vi "Update State on Cursor Move.vi"(9 "Cursor.Position.X":dbl, 10 "Cursor Name":string, 11 "Display State In":T1 caption="State") -> (2 "cursor type":string, 3 "Display State out":T1 caption="State")   [LabVIEW 2017, in "Waveforms with Cursors.xctl"]
uses:
  <vilib>/addons/_XControls/Waveforms with Cursors/Waveforms with Cursors.xctl
  <vilib>/addons/_XControls/Waveforms with Cursors/Controls/State.ctl
  <vilib>/Utility/miscctls.llb/LVFontTypeDef.ctl
  <vilib>/addons/_XControls/Waveforms with Cursors/Controls/Waveform Cursor Configuration.ctl
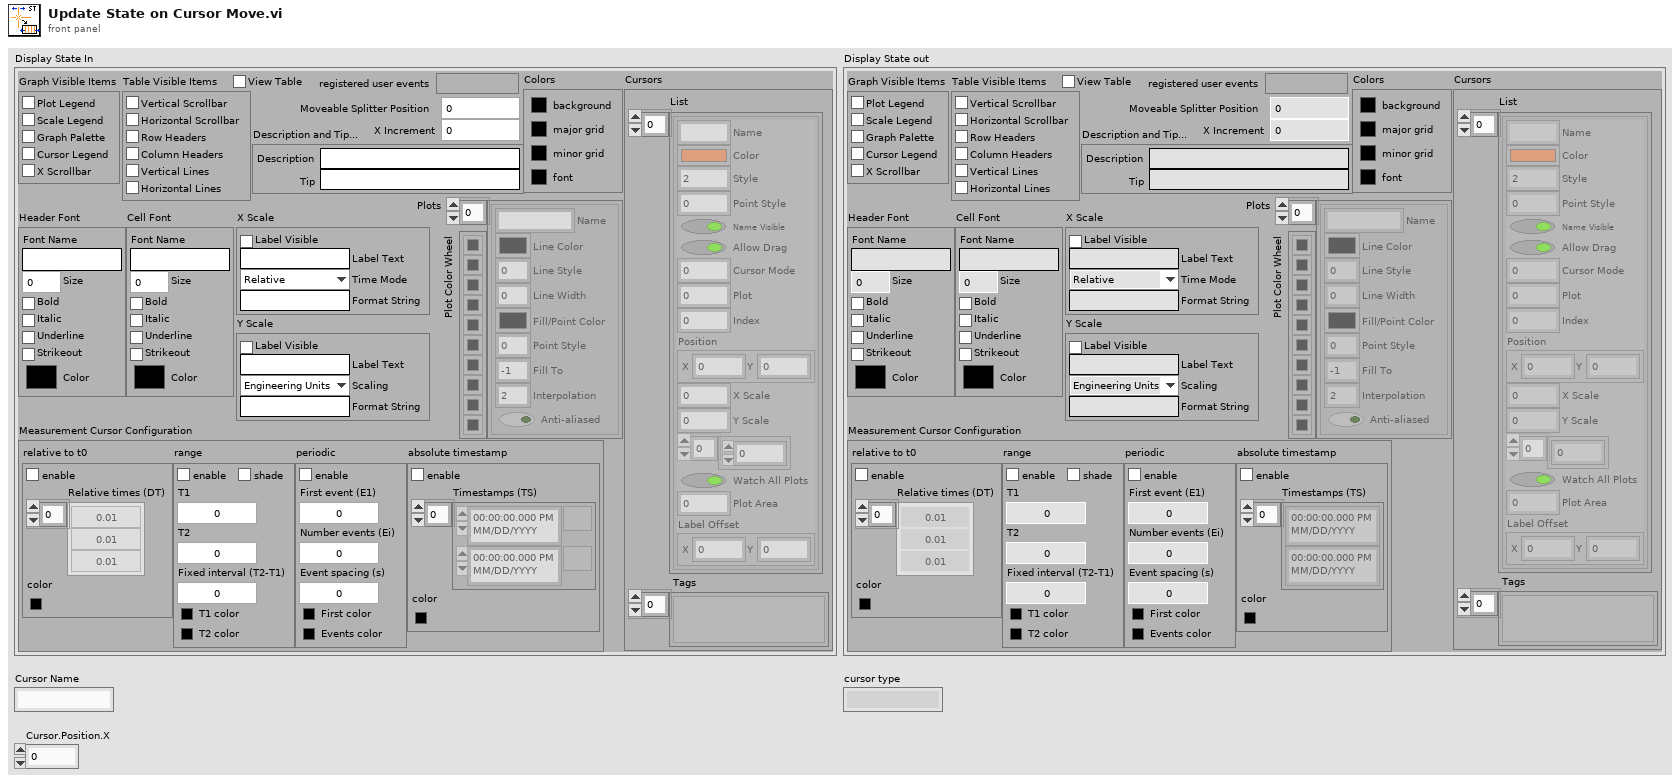
[diagram p1: front panel]
types:
  T1 = typedef "Waveforms with Cursors.xctl/State.ctl" = cluster{"Graph Visible Items":cluster{"Plot Legend":bool, "Scale Legend":bool, "Graph Palette":bool, "Cursor Legend":bool, "X Scrollbar":bool}, "View Table":bool, "Table Visible Items":cluster{"Vertical Scrollbar":bool, "Horizontal Scrollbar":bool, "Row Headers":bool, "Column Headers":bool, "Vertical Lines":bool, "Horizontal Lines":bool}, "Header Font":T2, "Cell Font":T2, "Description and Tip...":cluster{"Description":string, "Tip":string}, "Moveable Splitter Position":i32, "Measurement Cursor Configuration":T3, "X Increment":dbl, "X Scale":cluster{"Label Visible":bool, "Label Text":string, "Time Mode":enum16{"Relative", "Absolute"}, "Format String":string}, "Y Scale":cluster{"Label Visible":bool, "Label Text":string, "Scaling":enum16{"Engineering Units", "Voltage"}, "Format String":string}, "Colors":cluster{"background":u32, "major grid":u32, "minor grid":u32, "font":u32}, "Cursors":cluster{"List":cluster{"Name":string, "Color":u32, "Style":i32, "Point Style":u8, "Name Visible":bool, "Allow Drag":bool, "Cursor Mode":u32, "Plot":i32, "Index":i32, "Position":cluster{"X":dbl, "Y":dbl}, "X Scale":u32, "Y Scale":u32, "Watch Plots":i32[], "Watch All Plots":bool, "Plot Area":i32, "Label Offset":cluster{"X":dbl, "Y":dbl}}[], "Tags":variant[]}, "Plots":cluster{"Name":string, "Line Color":u32, "Line Style":u8, "Line Width":u8, "Fill/Point Color":u32, "Point Style":u8, "Fill To":i16, "Interpolation":u8, "Anti-aliased":bool}[], "Plot Color Wheel":u32[], "registered user events":variant}
  T2 = typedef "LVFontTypeDef.ctl" = cluster{"Font Name":string, "Size":u16, "Bold":bool, "Italic":bool, "Underline":bool, "Strikeout":bool, "Color":u32}
  T3 = typedef "Waveforms with Cursors.xctl/Waveform Cursor Configuration.ctl" = cluster{"relative to t0":cluster{"enable relative time":bool, "Relative times (DT)":dbl[], "color":u32}, "range":cluster{"enable range":bool, "T1":dbl, "T2":dbl, "Fixed interval (T2-T1)":dbl, "T1 color":u32, "T2 color":u32, "enable shading":bool}, "periodic":cluster{"enable periodic":bool, "First event (E1)":dbl, "Number events (Ei)":i32, "Event spacing (s)":dbl, "First color":u32, "Events color":u32}, "absolute timestamp":cluster{"enable absolute":bool, "Timestamps (TS)":timestamp[], "color":u32}}
  T4 = cluster{"Name":string, "Color":u32, "Style":i32, "Point Style":u8, "Name Visible":bool, "Allow Drag":bool, "Cursor Mode":u32, "Plot":i32, "Index":i32, "Position":cluster{"X":dbl, "Y":dbl}, "X Scale":u32, "Y Scale":u32, "Watch Plots":i32[], "Watch All Plots":bool, "Plot Area":i32, "Label Offset":cluster{"X":dbl, "Y":dbl}}[]
  T5 = cluster{"Name":string, "Color":u32, "Style":i32, "Point Style":u8, "Name Visible":bool, "Allow Drag":bool, "Cursor Mode":u32, "Plot":i32, "Index":i32, "Position":cluster{"X":dbl, "Y":dbl}, "X Scale":u32, "Y Scale":u32, "Watch Plots":i32[], "Watch All Plots":bool, "Plot Area":i32, "Label Offset":cluster{"X":dbl, "Y":dbl}}
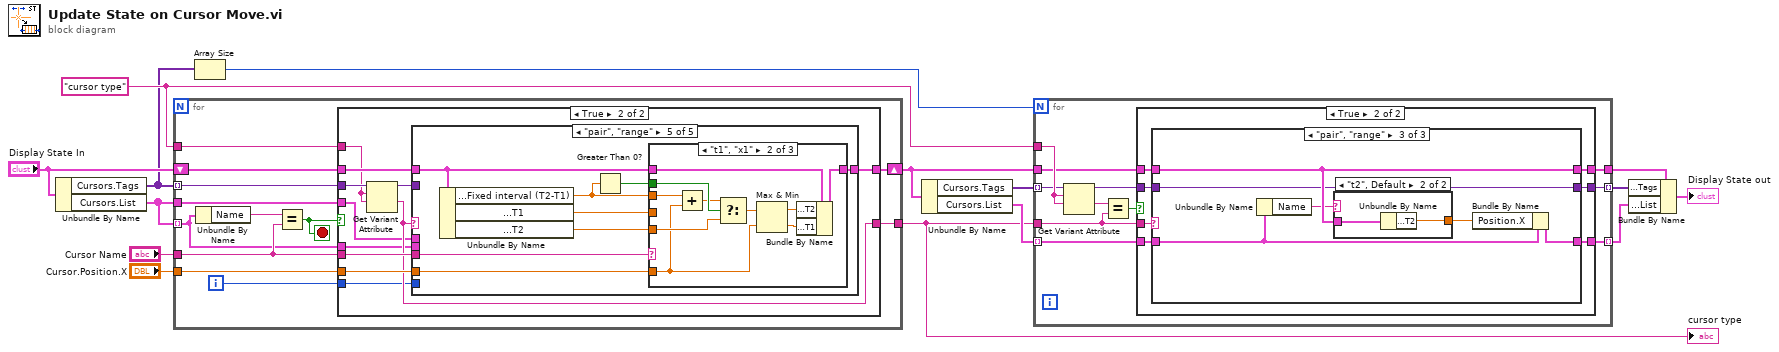
[diagram p0: block diagram]
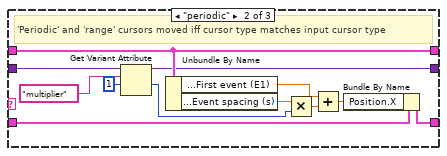
[diagram p4: hidden frame]
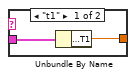
[diagram p5: hidden frame]
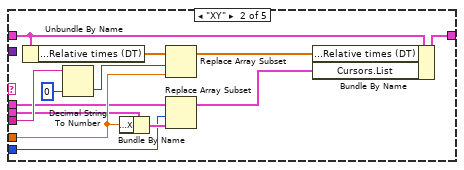
[diagram p8: hidden frame]
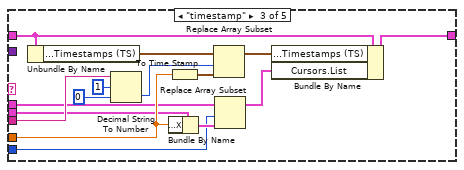
[diagram p9: hidden frame]
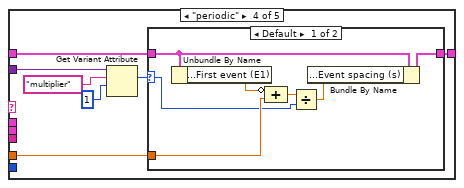
[diagram p10: hidden frame]
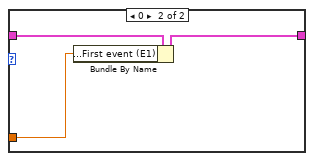
[diagram p11: hidden frame]
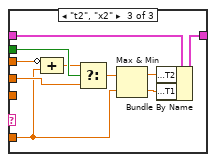
[diagram p13: hidden frame]
diagram:
  w12 = "cursor type"
  n1 = Unbundle By Name("Display State In") -> ("Cursors.Tags"=w2:variant[], "Cursors.List"=w4:T4)
  n2 = for {
    tunnel: "Cursor Name" -> [w24]
    tunnel: "Cursor.Position.X" -> [w25]
    shift-right: [w26] -> w14
    shift-left: "Display State In" -> [w27]
    tunnel: [w23] -> w5
    tunnel: w12 -> [w22]
    tunnel: w2 -> [w21] mode=indexing
    tunnel: w4 -> [w18] mode=indexing
    tunnel: w4 -> [w19]
    i -> [w17]
    stop <- w16 stop-if-true
    n3 = Unbundle By Name(w18) -> ("Name"=w20:string)
    n4 = Equal?(x=w20, y=w24) -> (x = y?=w16:bool)
    n5 = case shown="True" w16 {
      tunnel: w21 -> [_ w39]
      tunnel: w22 -> [_ w32]
      tunnel: w27 -> [w28 w38]
      tunnel: [w28 w37] -> w26
      tunnel: w25 -> [_ w35]
      tunnel: w24 -> [_ w34]
      tunnel: [_ w33] -> w23
      tunnel: w19 -> [_ w31]
      tunnel: w18 -> [_ w30]
      tunnel: w17 -> [_ w29]
      frame False {
      }
      frame True {
        n6 = Get Variant Attribute(Variant=w39, name=w32, default value (empty Variant)=w32) -> (duplicate Variant=w36:variant, value=w33:string)  [unwired: 1 in, 2 out]
        n7 = case shown="\"pair\", \"range\"" w33 {
          tunnel: w38 -> [w40 w51 w66 w75 w91]
          tunnel: [w40 w53 w68 w74 w93] -> w37
          tunnel: w36 -> [_ _ _ w73 _]
          tunnel: w35 -> [_ w46 w58 w70 w92]
          tunnel: w34 -> [_ w47 w62 _ w90]
          tunnel: w31 -> [_ w44 w56 _ _]
          tunnel: w30 -> [_ w45 w57 _ _]
          tunnel: w29 -> [_ w42 w55 _ _]
          frame Default {
          }
          frame "XY" {
            n8 = Unbundle By Name(w51) -> ("Measurement Cursor Configuration.relative to t0.Relative times (DT)"=w50:dbl[])
            n9 = Decimal String To Number(string=w47, default (0L)=0 ("default (0 I32)")) -> (number=w49:i32)  [unwired: 1 in, 1 out]
            n10 = Bundle By Name(cluster=w45, "Position.X"=w46) -> (w43:T5)
            n11 = Replace Array Subset(array=w50, new element=w46, index=w49) -> (w48:dbl[])
            n12 = Replace Array Subset(array=w44, new element=w43, index=w42) -> (w41:T4)
            n13 = Bundle By Name(cluster=w51, "Measurement Cursor Configuration.relative to t0.Relative times (DT)"=w48, "Cursors.List"=w41) -> (w53:T1)
          }
          frame "timestamp" {
            n14 = Unbundle By Name(w66) -> ("Measurement Cursor Configuration.absolute timestamp.Timestamps (TS)"=w65:timestamp[])
            n15 = Decimal String To Number(string=w62, offset=1, default (0L)=0 ("default (0 I32)")) -> (number=w64:i32)  [unwired: 1 out]
            n16 = Bundle By Name(cluster=w57, "Position.X"=w58) -> (w59:T5)
            n17 = To Time Stamp(1:w58) -> (0:w61:timestamp)
            n18 = Replace Array Subset(array=w65, new element=w61, index=w64) -> (w63:timestamp[])
            n19 = Replace Array Subset(array=w56, new element=w59, index=w55) -> (w54:T4)
            n20 = Bundle By Name(cluster=w66, "Measurement Cursor Configuration.absolute timestamp.Timestamps (TS)"=w63, "Cursors.List"=w54) -> (w68:T1)
          }
          frame "periodic" {
            n21 = Get Variant Attribute(Variant=w73, name="multiplier", default value (empty Variant)=1) -> (value=w69:i32)  [unwired: 1 in, 3 out]
            n22 = case shown="Default" w69 {
              selector: w69 -> [w78 _]
              tunnel: w75 -> [w81 w85]
              tunnel: [w82 w84] -> w74
              tunnel: w70 -> [w79 w83]
              frame Default {
                n23 = Unbundle By Name(w81) -> ("Measurement Cursor Configuration.periodic.First event (E1)"=w80:dbl)
                n24 = Compound Arithmetic op=ADD(invert w80, w79) -> (w77:dbl)
                n25 = Divide(x=w77, y=w78) -> (x/y=w76:dbl)
                n26 = Bundle By Name(cluster=w81, "Measurement Cursor Configuration.periodic.Event spacing (s)"=w76) -> (w82:T1)
              }
              frame 0 {
                n27 = Bundle By Name(cluster=w85, "Measurement Cursor Configuration.periodic.First event (E1)"=w83) -> (w84:T1)
              }
            }
          }
          frame "pair", "range" {
            n28 = Unbundle By Name(w91) -> ("Measurement Cursor Configuration.range.Fixed interval (T2-T1)"=w86:dbl, "Measurement Cursor Configuration.range.T1"=w89:dbl, "Measurement Cursor Configuration.range.T2"=w88:dbl)
            n29 = Greater Than 0?(x=w86) -> (x > 0?=w87:bool)
            n30 = case shown="\"t1\", \"x1\"" w90 {
              tunnel: w91 -> [w94 w104 w114]
              tunnel: [w94 w103 w113] -> w93
              tunnel: w92 -> [_ w97 w105]
              tunnel: w89 -> [_ _ w106]
              tunnel: w88 -> [_ w99 _]
              tunnel: w86 -> [_ w101 w111]
              tunnel: w87 -> [_ w102 w112]
              frame Default {
              }
              frame "t1", "x1" {
                n31 = Add(x=w101, y=w97) -> (x+y=w100:dbl)
                n32 = Select(t=w100, s=w102, f=w99) -> (s? t:f=w98:dbl)
                n33 = Max & Min(x=w98, y=w97) -> (max(x,y)=w96:dbl, min(x,y)=w95:dbl)
                n34 = Bundle By Name(cluster=w104, "Measurement Cursor Configuration.range.T2"=w96, "Measurement Cursor Configuration.range.T1"=w95) -> (w103:T1)
              }
              frame "t2", "x2" {
                n35 = Compound Arithmetic op=ADD(invert w111, w105) -> (w110:dbl)
                n36 = Select(t=w110, s=w112, f=w106) -> (s? t:f=w109:dbl)
                n37 = Max & Min(x=w109, y=w105) -> (max(x,y)=w108:dbl, min(x,y)=w107:dbl)
                n38 = Bundle By Name(cluster=w114, "Measurement Cursor Configuration.range.T2"=w108, "Measurement Cursor Configuration.range.T1"=w107) -> (w113:T1)
              }
            }
          }
        }
      }
    }
  }
  "cursor type" <- w5
  n39 = Array Size(array=w2) -> (size(s)=w3:i32)
  n40 = Unbundle By Name(w14) -> ("Cursors.Tags"=w6:variant[], "Cursors.List"=w7:T4)
  n41 = for {
    N: w3 -> [_]
    tunnel: w12 -> [w125]
    tunnel: w5 -> [w121]
    tunnel: w6 -> [w119] mode=indexing
    tunnel: w7 -> [w118] mode=indexing
    tunnel: w14 -> [w120]
    tunnel: [w117] -> w8 mode=indexing
    tunnel: [w116] -> w9 mode=indexing
    tunnel: [w115] -> w10
    n42 = Get Variant Attribute(Variant=w119, name=w125, default value (empty Variant)=w125) -> (duplicate Variant=w124:variant, value=w122:string)  [unwired: 1 in, 2 out]
    n43 = Equal?(x=w122, y=w121) -> (x = y?=w123:bool)
    n44 = case shown="True" w123 {
      tunnel: w124 -> [w127 w133]
      tunnel: w120 -> [w128 w135]
      tunnel: w121 -> [_ w134]
      tunnel: [w128 w132] -> w115
      tunnel: w118 -> [w126 w131]
      tunnel: [w126 w130] -> w117
      tunnel: [w127 w129] -> w116
      frame False {
      }
      frame True {
        n45 = case shown="\"pair\", \"range\"" w134 {
          tunnel: w135 -> [w138 w141 w156]
          tunnel: w133 -> [w137 w150 w155]
          tunnel: [w138 w141 w156] -> w132
          tunnel: w131 -> [w136 w142 w153]
          tunnel: [w136 w140 w154] -> w130
          tunnel: [w137 w139 w155] -> w129
          frame Default {
            # "'XY' and 'timestamp' cursors are moved individually rather than as set"
          }
          frame "periodic" {
            # "'Periodic' and 'range' cursors moved iff cursor type matches input cursor type"
            n46 = Get Variant Attribute(Variant=w150, name="multiplier", default value (empty Variant)=1) -> (duplicate Variant=w139:variant, value=w145:i32)  [unwired: 1 in, 2 out]
            n47 = Unbundle By Name(w141) -> ("Measurement Cursor Configuration.periodic.First event (E1)"=w146:dbl, "Measurement Cursor Configuration.periodic.Event spacing (s)"=w147:dbl)
            n48 = Multiply(x=w147, y=w145) -> (x*y=w144:dbl)
            n49 = Add(x=w146, y=w144) -> (x+y=w143:dbl)
            n50 = Bundle By Name(cluster=w142, "Position.X"=w143) -> (w140:T5)
          }
          frame "pair", "range" {
            n51 = Unbundle By Name(w153) -> ("Name"=w152:string)
            n52 = case shown="\"t2\", Default" w152 {
              tunnel: w156 -> [w158 w160]
              tunnel: [w157 w159] -> w151
              frame "t1" {
                n53 = Unbundle By Name(w158) -> ("Measurement Cursor Configuration.range.T1"=w157:dbl)
              }
              frame "t2", Default {
                n54 = Unbundle By Name(w160) -> ("Measurement Cursor Configuration.range.T2"=w159:dbl)
              }
            }
            n55 = Bundle By Name(cluster=w153, "Position.X"=w151) -> (w154:T5)
          }
        }
      }
    }
  }
  n56 = Bundle By Name(cluster=w10, "Cursors.Tags"=w9, "Cursors.List"=w8) -> (→"Display State out":T1)
